vi "EDS Read.vi"(11 "SDO Parameters":T1[](array[typedef]) {"Sub-Index (0)" format="%.0x"; "Object Index" format="%.0x"; "Block Data" format="%.0x"}) -> (3 "SDO Parameters out":T1[](array[typedef]) {"Sub-Index (0)" format="%.0x"; "Object Index" format="%.0x"; "Block Data" format="%.0x"})   [LabVIEW 2021, in "CANOpen Addon System Explorer.lvlib"]
uses:
  CANOpen Addon System Explorer.lvlib
  control/Data.ctl
  control/File Information.ctl
  control/Dummy Usage.ctl
  control/OD Entry.ctl
  control/Object Type.ctl
  control/Data Type.ctl
  control/Access Type.ctl
  control/OD Cateory.ctl
  Shared/CANOpen_SDO Settings.ctl
  silver control/Silver Status.ctl
  Shared/CANOpen Addon Shared.lvlib
panel:
  out "Loading":string="Loading EDS file. Please wait!"
  in  "Cancel Button":bool
  in  "OK Button":bool
  in  "EDS Tree":string[](tree)
  in  "EDS Data":T2={"FileInfo"={"FileName"="", "FileVersion"=0, "FileRevision"=0, "EDSVersion"="4.0", "Description"="", "CreationTime"=0.0, "CreationDate"=0.0, "CreatedBy"="", "ModificationTime"=0.0, "ModificationDate"=0.0, "ModifiedBy"=""}, "DeviceInfo"={"Bitfile Name"=path "", "Signature"=[], "Control Offsets"={"StartCtrlOffset"=0, "LoopRateCtrlOffset"=0, "ExternalTimedCtrlOffset"=0, "RTSICtrlOffset"=0, "GenIRQCtrlOffset"=0, "HWSynchCtrlOffset"=0}, "DMA Offsets"={"ReadDMAOffset"=0, "WriteDMAOffset"=0}, "Buffer Sizes"={"NumReadPackets"=0, "NumWritePackets"=0, "NumberOfReadChannels"=0, "NumberOfWriteChannels"=0}}, "DummyUsage"={"Dummy0001"=FALSE, "Dummy0002"=FALSE, "Dummy0003"=FALSE, "Dummy0004"=FALSE, "Dummy0005"=FALSE, "Dummy0006"=FALSE, "Dummy0007"=FALSE}, "OD Entries"=[]} {"OD Entries"."SubNumber" format="%x"; "OD Entries"."AccessType" items=["", "ro", "wo", "rw", "const", "rwr", "rww"]; "OD Entries"."DataType" items=[""=0, "BOOLEAN"=1, "INTEGER8"=2, "INTEGER16"=3, "INTEGER32"=4, "UNSIGNED8"=5, "UNSIGNED16"=6, "UNSIGNED32"=7, "REAL32"=8, "VISIBLE_STRING"=9, "OCTET_STRING"=10, "UNICODE_STRING"=11, "TIME_OF_DAY"=12, "TIME_DIFFERENCE"=13, "DOMAIN"=15, "INTEGER24"=16, "REAL64"=17, "INTEGER40"=18, "INTEGER48"=19, "INTEGER56"=20, "INTEGER64"=21, "UNSIGNED24"=22, "UNSIGNED40"=24, "UNSIGNED48"=25, "UNSIGNED56"=26, "UNSIGNED64"=27]; "OD Entries"."ObjectType" items=[""=10, "NULL"=0, "DOMAIN"=2, "DEFTYPE"=5, "DEFSTRUCT"=6, "VAR"=7, "ARRAY"=8, "RECORD"=9]; "OD Entries"."sub-index" format="%x"; "OD Entries"."index" format="%x"; "FileInfo"."ModificationDate" format="%<%m-%d-%Y>T"; "FileInfo"."ModificationTime" format="%<%I:%M%p>T"; "FileInfo"."CreationDate" format="%<%m-%d-%Y>T"; "FileInfo"."CreationTime" format="%<%I:%M%p>T"}
  in  "EDS File Path":path
  # "LSB"
  # "MSB"
  # "LSB"
  # "MSB"
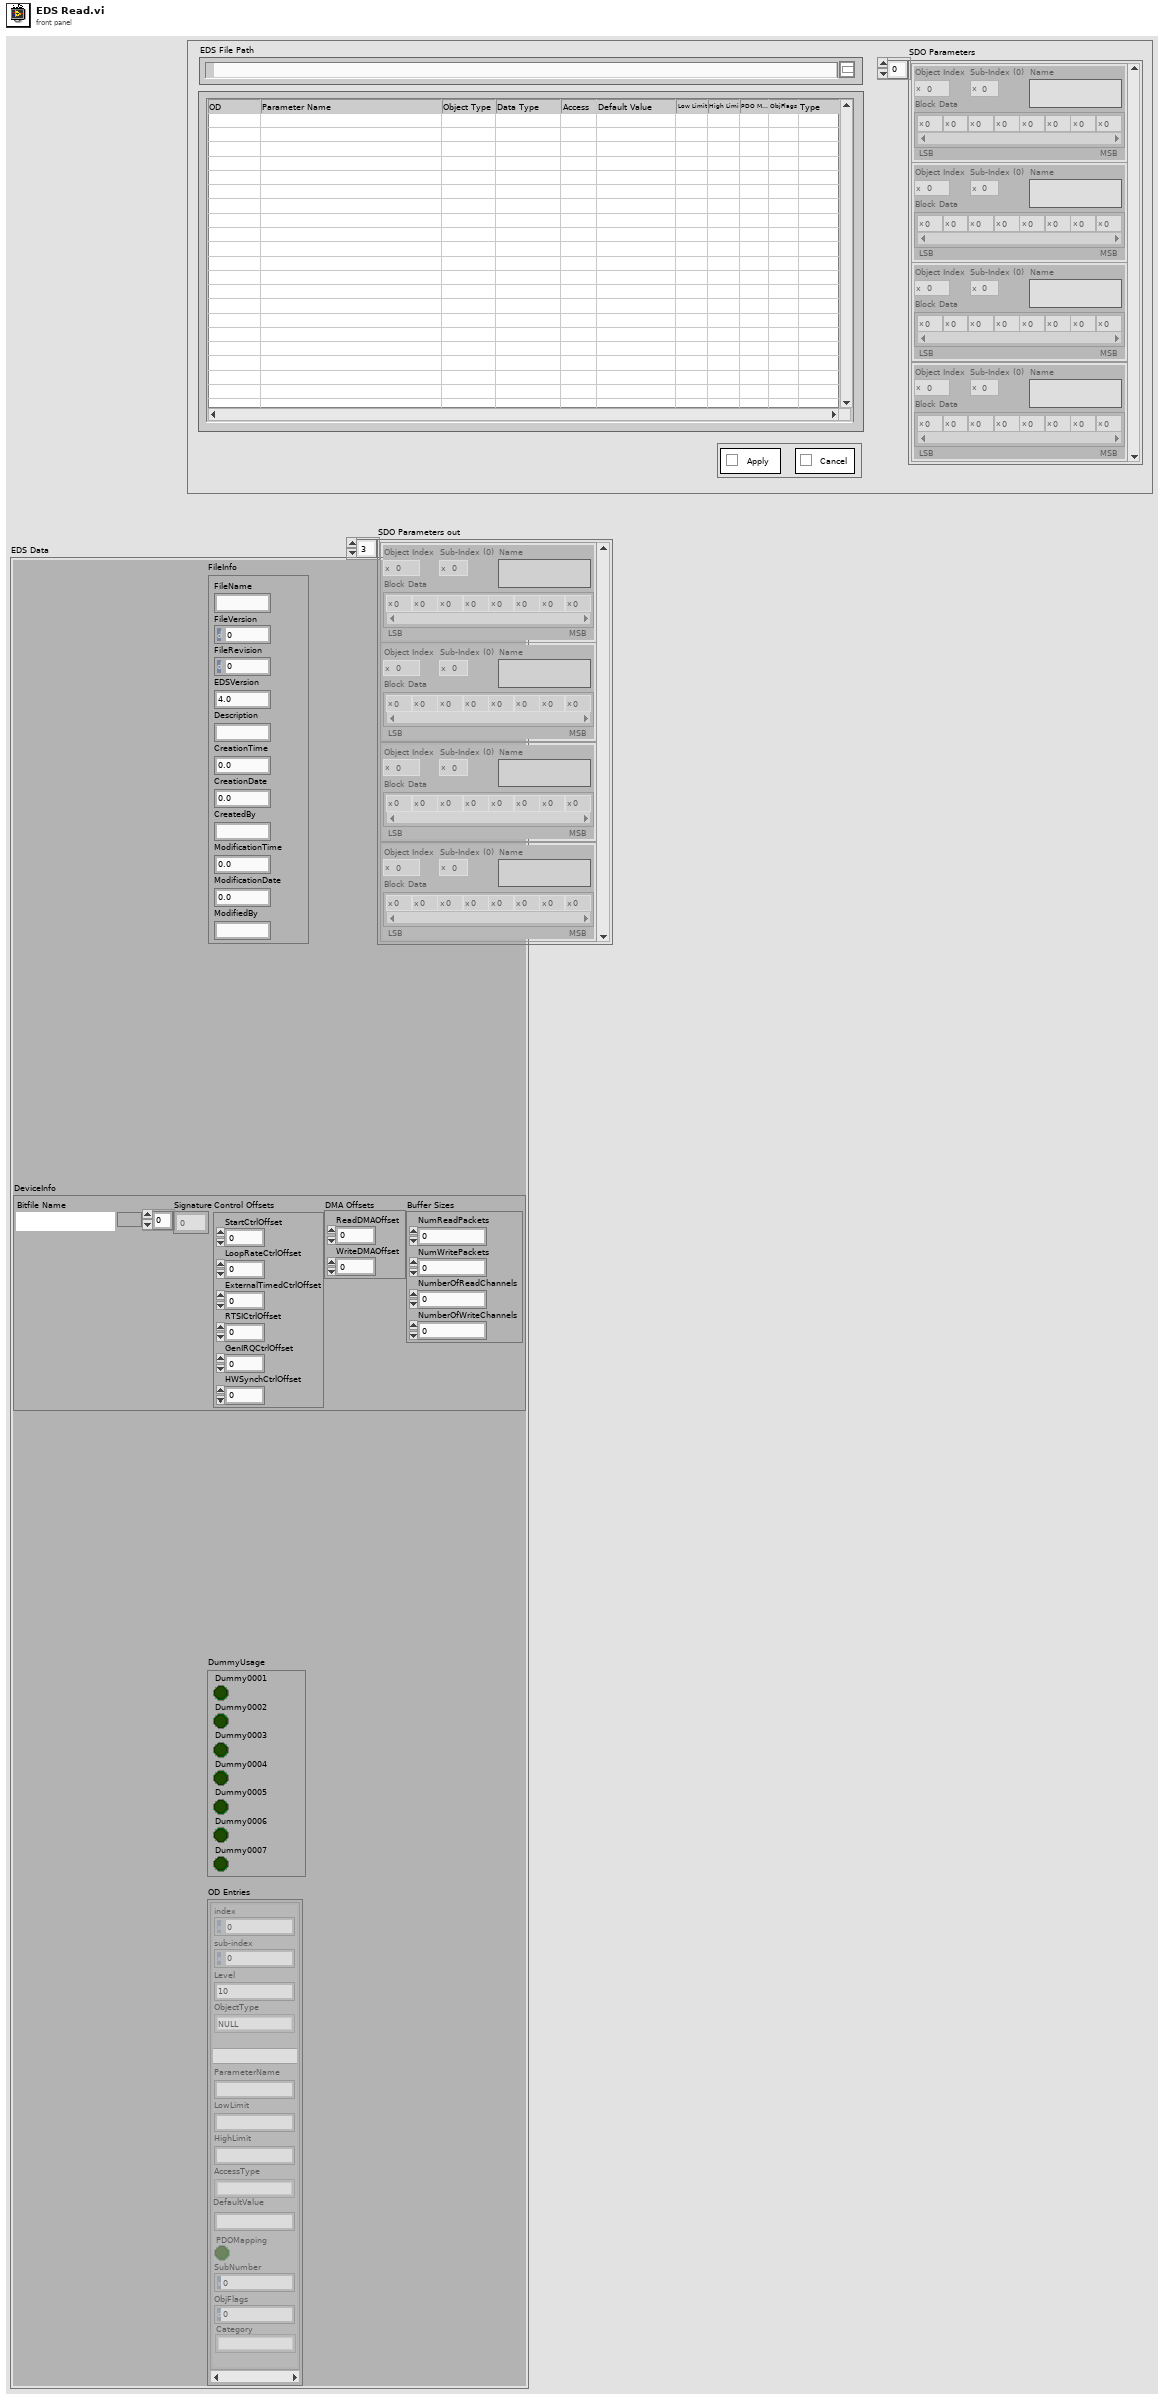
[diagram p1: front panel]
types:
  T1 = typedef "CANOpen Addon Shared.lvlib/CANOpen_SDO Settings.ctl" = cluster{"Object Index":u16, "Sub-Index (0)":u8, "Block Data":u8[], "Name":string}
  T2 = typedef "CANOpen Addon System Explorer.lvlib/Data.ctl" = cluster{"FileInfo":T3, "DeviceInfo":cluster{"Bitfile Name":path, "Signature":u8[], "Control Offsets":cluster{"StartCtrlOffset":u32, "LoopRateCtrlOffset":u32, "ExternalTimedCtrlOffset":u32, "RTSICtrlOffset":u32, "GenIRQCtrlOffset":u32, "HWSynchCtrlOffset":u32}, "DMA Offsets":cluster{"ReadDMAOffset":u32, "WriteDMAOffset":u32}, "Buffer Sizes":cluster{"NumReadPackets":u32, "NumWritePackets":u32, "NumberOfReadChannels":u32, "NumberOfWriteChannels":u32}}, "DummyUsage":T4, "OD Entries":T5[]}
  T3 = typedef "CANOpen Addon System Explorer.lvlib/File Information.ctl" = cluster{"FileName":string, "FileVersion":u8, "FileRevision":u8, "EDSVersion":string, "Description":string, "CreationTime":dbl, "CreationDate":dbl, "CreatedBy":string, "ModificationTime":dbl, "ModificationDate":dbl, "ModifiedBy":string}
  T4 = typedef "CANOpen Addon System Explorer.lvlib/Dummy Usage.ctl" = cluster{"Dummy0001":bool, "Dummy0002":bool, "Dummy0003":bool, "Dummy0004":bool, "Dummy0005":bool, "Dummy0006":bool, "Dummy0007":bool}
  T5 = typedef "CANOpen Addon System Explorer.lvlib/OD Entry.ctl" = cluster{"index":u16, "sub-index":u8, "Level":u8, "ObjectType":T6, "DataType":T7, "ParameterName":string, "LowLimit":string, "HighLimit":string, "AccessType":T8, "DefaultValue":string, "PDOMapping":bool, "SubNumber":u8, "ObjFlags":u32, "Category":T9}
  T6 = typedef "CANOpen Addon System Explorer.lvlib/Object Type.ctl" = u16
  T7 = typedef "CANOpen Addon System Explorer.lvlib/Data Type.ctl" = u16
  T8 = typedef "CANOpen Addon System Explorer.lvlib/Access Type.ctl" = u16
  T9 = typedef "CANOpen Addon System Explorer.lvlib/OD Cateory.ctl" = enum16{"Mandatory", "Optional", "Manufacturer", ""}
  T10 = typedef "CANOpen Addon System Explorer.lvlib/Silver Status.ctl" = enum16{"Idle", "Initial", "Open EDS", "Display EDS OD", "Shutdown"}
  T11 = cluster{"index":u16, "sub-index":u8, "Level":u8, "ObjectType":T6, "DataType":T7, "ParameterName":string, "DefaultValue":string, "SubNumber":u8}
  T12 = enum8{"Enabled", "Disabled", "Disabled and Grayed Out"}
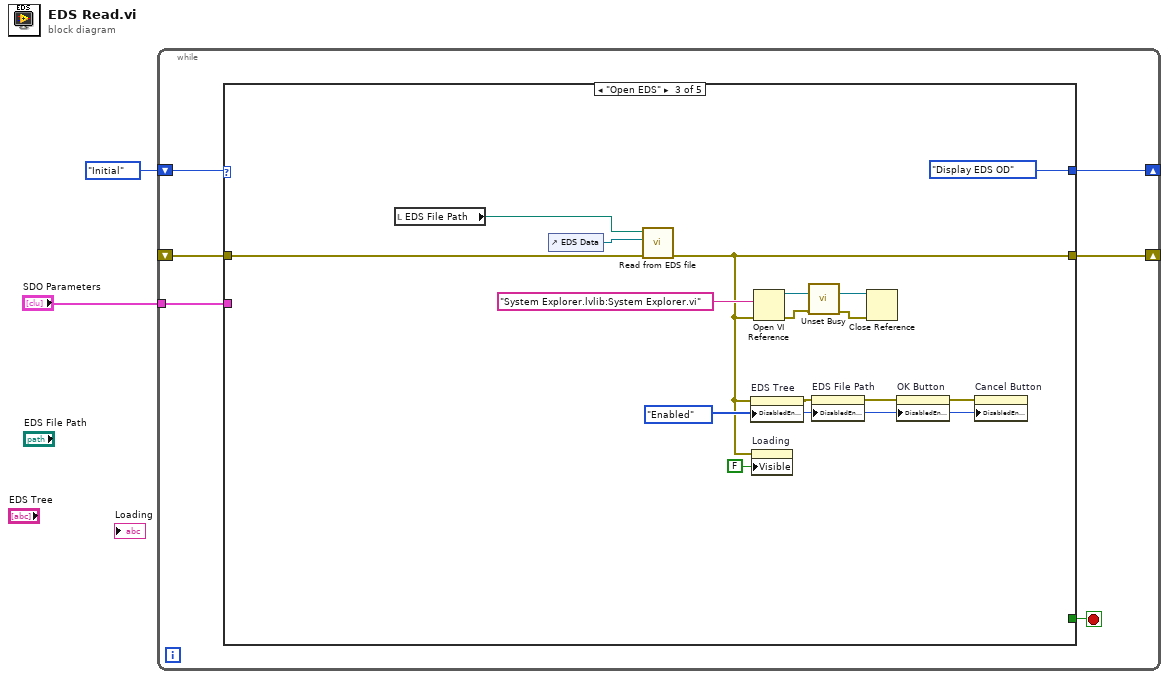
[diagram p0: block diagram]
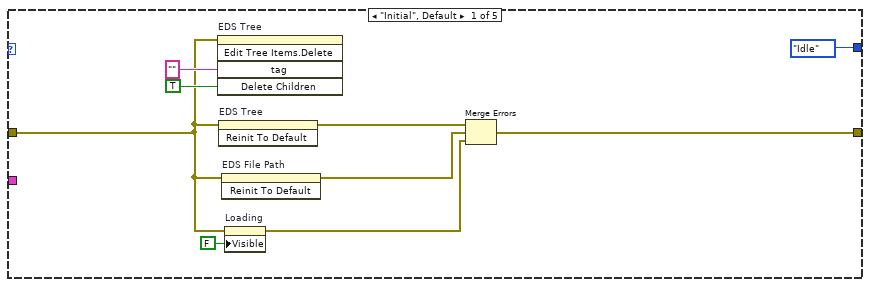
[diagram p2: hidden frame]
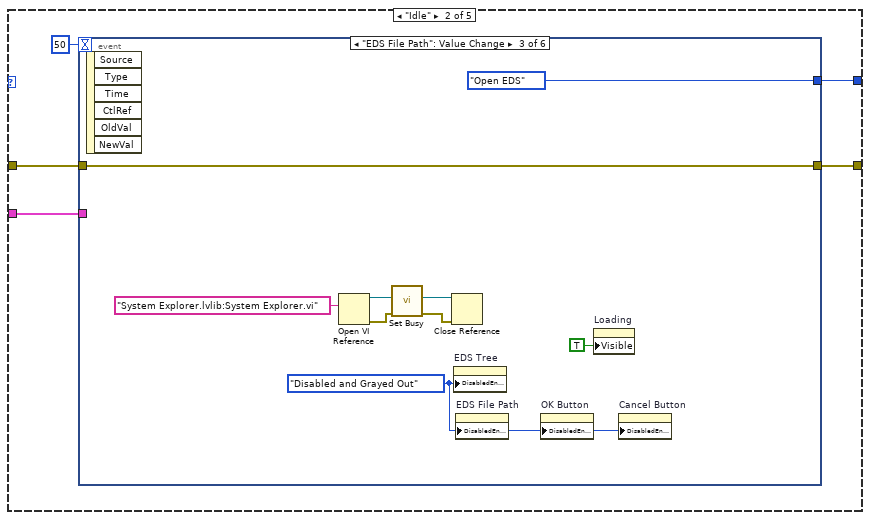
[diagram p3: hidden frame]
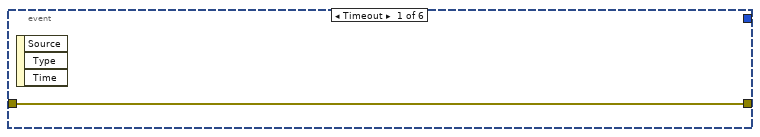
[diagram p4: hidden frame]
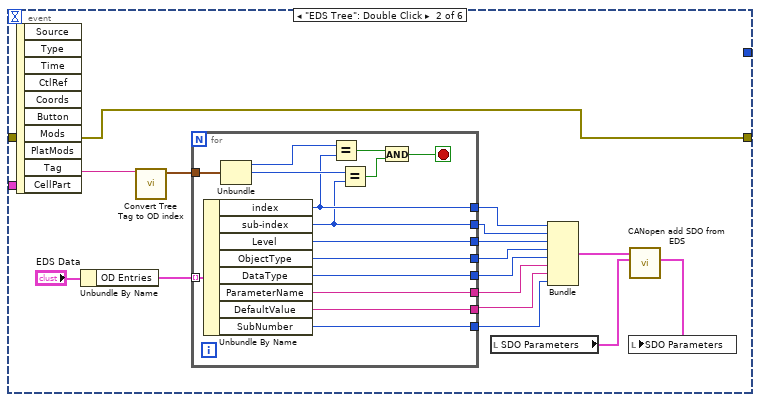
[diagram p5: hidden frame]
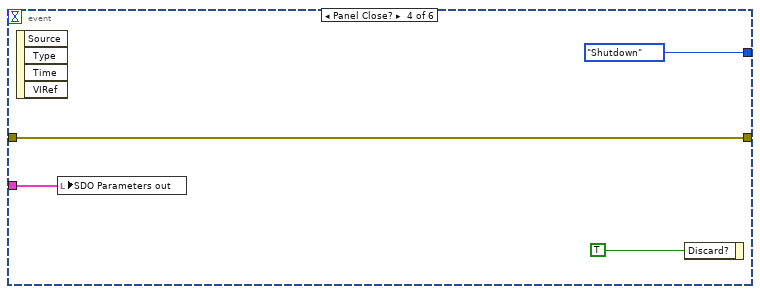
[diagram p6: hidden frame]
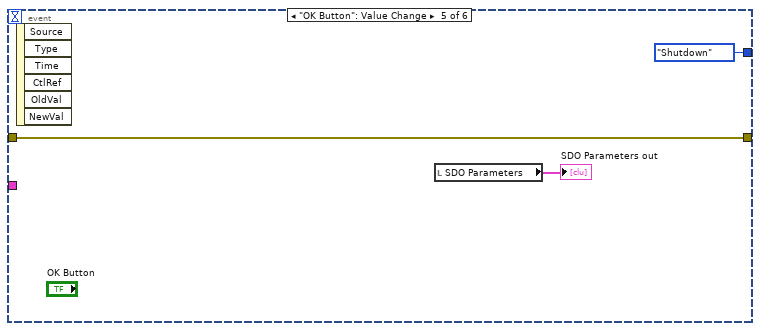
[diagram p7: hidden frame]
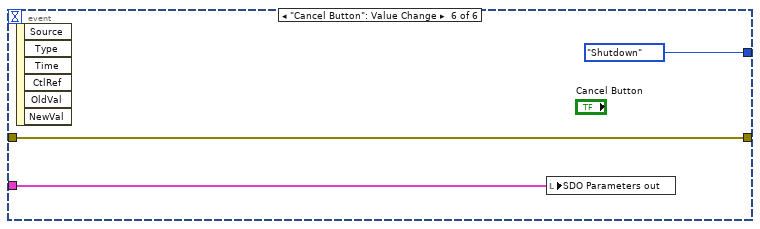
[diagram p8: hidden frame]
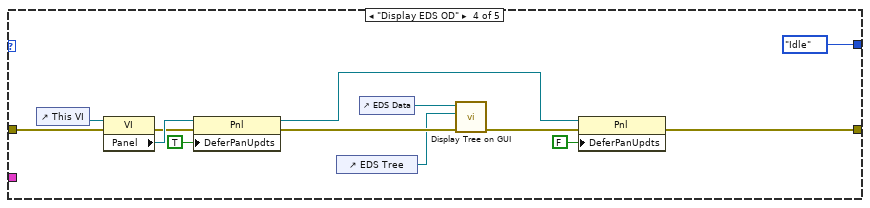
[diagram p9: hidden frame]
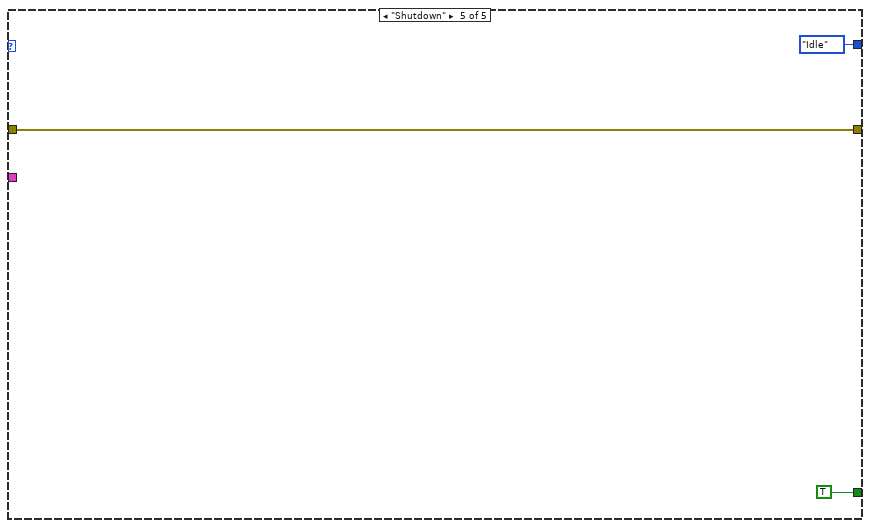
[diagram p10: hidden frame]
diagram:
  n1 = while {
    shift-right: [w7] -> _
    shift-left: _ -> [w8]
    shift-right: [w6] -> _
    shift-left: Silver_Status."Initial" ("Enum") -> [w5]
    tunnel: "SDO Parameters" -> [w3]
    stop <- w4 stop-if-true
    n2 = case shown="\"Open EDS\"" w5 {
      tunnel: w8 -> [w10 w18 w83 w96 w100]
      tunnel: [w12 w19 w73 w91 w100] -> w7
      tunnel: [Silver_Status."Idle" ("Enum") w22 Silver_Status."Display EDS OD" ("Enum") Silver_Status."Idle" ("Enum") Silver_Status."Idle" ("Enum")] -> w6
      tunnel: [_ _ _ _ TRUE] -> w4
      tunnel: w3 -> [_ w20 _ _ _]
      frame "Initial", Default {
        n3 = invoke on="EDS Tree" class="Tree (strict)" method="Edit Tree Items.Delete"(error in=w10, "tag"="" ("Tag"), "Delete Children"=TRUE ("Delete Children?")) -> ()  [unwired: 2 in, 5 out]
        n4 = invoke on="EDS Tree" class="Tree (strict)" method="Reinit To Default"(error in=w10) -> (error out=w14:errorcluster)  [unwired: 2 in, 2 out]
        n5 = invoke on="EDS File Path" class="Path" method="Reinit To Default"(error in=w10) -> (error out=w13:errorcluster)  [unwired: 2 in, 2 out]
        n6 = property on="Loading" class="Str"(error in=w10, "Visible"=FALSE) -> (error out=w9:errorcluster)  [unwired: 1 in, 1 out]
        n7 = Merge Errors(w14, w13, w9) -> (w12:errorcluster)
      }
      frame "Idle" {
        n8 = event shown="[2] \"EDS File Path\": Value Change" {
          selector: _ -> [_ _ _ _ _ _]
          dyn-events: _ -> [_ _ _ _ _ _]
          timeout: 50 -> [_ _ _ _ _ _]
          tunnel: [_ _ Silver_Status."Open EDS" ("Enum") Silver_Status."Shutdown" ("Enum") Silver_Status."Shutdown" ("Enum") Silver_Status."Shutdown" ("Enum")] -> w22
          tunnel: w20 -> [_ _ _ w64 _ w71]
          tunnel: [w23 w27 w61 w63 w67 w70] -> w19
          tunnel: w18 -> [w23 w27 w61 w63 w67 w70]
          event Timeout {
            n9 = event-data() -> ()  [unwired: 1 in, 3 out]
          }
          event "EDS Tree": Double Click {
            n10 = event-data() -> ("Tag"=w30:string)  [unwired: 1 in, 9 out]
            n11 = Unbundle By Name("EDS Data") -> ("OD Entries"=w38:T5[])
            n12 = call "Convert Tree Tag to OD index.vi"("Tag"=w30) -> ("index"=w37:cluster{u16, u8, u8})  [unwired: 9 in, 1 out]
            n13 = for {
              tunnel: w38 -> [w54] mode=indexing
              tunnel: w37 -> [w53]
              tunnel: [w47] -> w36
              tunnel: [w46] -> w35
              tunnel: [w45] -> w34
              tunnel: [w44] -> w33
              tunnel: [w43] -> w32
              tunnel: [w42] -> w31
              tunnel: [w41] -> w29
              tunnel: [w40] -> w28
              stop <- w48 stop-if-true
              n14 = Unbundle By Name(w54) -> ("index"=w41:u16, "sub-index"=w40:u8, "Level"=w47:u8, "ObjectType"=w46:T6, "DataType"=w45:T7, "ParameterName"=w44:string, "DefaultValue"=w43:string, "SubNumber"=w42:u8)
              n15 = Unbundle(w53) -> (w52:u16, w51:u8)  [unwired: 1 out]
              n16 = Equal?(x=w52, y=w41) -> (x = y?=w50:bool)
              n17 = Equal?(x=w51, y=w40) -> (x = y?=w49:bool)
              n18 = And(x=w50, y=w49) -> (x .and. y?=w48:bool)
            }
            n19 = local read "SDO Parameters"() -> (w25:T1[])
            n20 = Bundle("index"=w29, "sub-index"=w28, "Level"=w36, "ObjectType"=w35, "DataType"=w34, "ParameterName"=w33, "DefaultValue"=w32, "SubNumber"=w31) -> (w26:T11)  [unwired: 1 in]
            n21 = call "CANopen add SDO from EDS.vi"("SDO Parameters in"=w25, "Cluster"=w26) -> ("SDO Parameters"=w24:T1[])  [unwired: 9 in]
            n22 = local write "SDO Parameters"(w24) -> ()
          }
          event "EDS File Path": Value Change {
            w56 = T12."Disabled and Grayed Out" ("Disabled")
            n23 = event-data() -> ()  [unwired: 1 in, 6 out]
            n24 = Open VI Reference(vi path="System Explorer.lvlib:System Explorer.vi" ("Separator (,)")) -> (vi reference=w58:refnum<vi>, error out=w59:errorcluster)  [unwired: 5 in]
            n25 = call <vilib>:"Set Busy.vi"("error in (no error)"=w59, "VI reference (current VI)"=w58) -> ("error out"=w57:errorcluster)  [unwired: 8 in, 1 out]
            n26 = Close Reference(reference=w58, error in (no error)=w57) -> ()  [unwired: 1 out]
            n27 = property on="EDS Tree" class="Tree (strict)"("DisabledEnum"=w56) -> ()  [unwired: 2 in, 2 out]
            n28 = property on="EDS File Path" class="Path"("DisabledEnum"=w56) -> ()  [unwired: 2 in, 2 out]
            n29 = property on="OK Button" class="Bool"("DisabledEnum"=w56) -> ()  [unwired: 2 in, 2 out]
            n30 = property on="Loading" class="Str"("Visible"=TRUE) -> ()  [unwired: 2 in, 2 out]
            n31 = property on="Cancel Button" class="Bool"("DisabledEnum"=w56) -> ()  [unwired: 2 in, 2 out]
          }
          event Panel Close? {
            n32 = event-data() -> ()  [unwired: 1 in, 4 out]
            n33 = local write "SDO Parameters out"(w64) -> ()
            n34 = event-data("Discard?"=TRUE) -> ()  [unwired: 1 in, 1 out]
          }
          event "OK Button": Value Change {
            n35 = event-data() -> ()  [unwired: 1 in, 6 out]
            n36 = local read "SDO Parameters"() -> (→"SDO Parameters out":T1[])
          }
          event "Cancel Button": Value Change {
            n37 = event-data() -> ()  [unwired: 1 in, 6 out]
            n38 = local write "SDO Parameters out"(w71) -> ()
          }
        }
      }
      frame "Open EDS" {
        w78 = T12."Enabled" ("Disabled")
        n39 = local read "EDS File Path"() -> (w86:path)
        n40 = control-ref of="EDS Data"() -> (w85:refnum<vi>)
        n41 = call "Read from EDS file.vi"("error in (no error)"=w83, "Clust Refnum"=w85, "EDS File Path"=w86) -> ("error out"=w73:errorcluster)  [unwired: 8 in]
        n42 = property on="EDS Tree" class="Tree (strict)"(error in=w73, "DisabledEnum"=w78) -> (error out=w76:errorcluster)  [unwired: 1 in, 1 out]
        n43 = property on="Loading" class="Str"(error in=w73, "Visible"=FALSE) -> ()  [unwired: 1 in, 2 out]
        n44 = Open VI Reference(vi path="System Explorer.lvlib:System Explorer.vi" ("Separator (,)"), error in (no error)=w73) -> (vi reference=w81:refnum<vi>, error out=w80:errorcluster)  [unwired: 4 in]
        n45 = call <vilib>:"Unset Busy.vi"("error in (no error)"=w80, "VI reference (current VI)"=w81) -> ("error out"=w79:errorcluster)  [unwired: 9 in]
        n46 = property on="EDS File Path" class="Path"(error in=w76, "DisabledEnum"=w78) -> (error out=w77:errorcluster)  [unwired: 1 in, 1 out]
        n47 = Close Reference(reference=w81, error in (no error)=w79) -> ()  [unwired: 1 out]
        n48 = property on="OK Button" class="Bool"(error in=w77, "DisabledEnum"=w78) -> (error out=w75:errorcluster)  [unwired: 1 in, 1 out]
        n49 = property on="Cancel Button" class="Bool"(error in=w75, "DisabledEnum"=w78) -> ()  [unwired: 1 in, 2 out]
      }
      frame "Display EDS OD" {
        n50 = control-ref of="This VI"() -> (w98:refnum<vi>)
        n51 = property class="VI"(reference=w98, error in=w96) -> (error out=w94:errorcluster, "Panel"=w97:refnum<vi>)  [unwired: 1 out]
        n52 = property class="Pnl"(reference=w97, error in=w94, "DeferPanUpdts"=TRUE ("Defer Panel Updates")) -> (reference out=w89:refnum<vi>, error out=w93:errorcluster)
        n53 = control-ref of="EDS Tree"() -> (w87:refnum<vi>)
        n54 = control-ref of="EDS Data"() -> (w99:refnum<vi>)
        n55 = call "Display Tree on GUI.vi"("error in (no error)"=w93, "Tree on GUI"=w87, "Data"=w99) -> ("error out"=w92:errorcluster)  [unwired: 8 in]
        n56 = property class="Pnl"(reference=w89, error in=w92, "DeferPanUpdts"=FALSE ("Defer Panel Updates")) -> (error out=w91:errorcluster)  [unwired: 1 out]
      }
      frame "Shutdown" {
      }
    }
  }
